vi "Check_Test_Voltage_and_Adjust.vi"(8 "error in":errorcluster, 11 "Voltage Desired":dbl format="%.6g") -> (0 "error out":errorcluster, 2 "Adjusted Voltage":dbl format="%.6g", 5 "Voltage Adjusted":bool)   [LabVIEW 2020]
uses:
  <vilib>/express/express arith-compare/Formula/XNode/ExpressFormulaBlockNode.xnode
panel:
  out "Outer While":i32
  out "Inner While":i32
  in  "Sample 1":dbl format="%.6g"
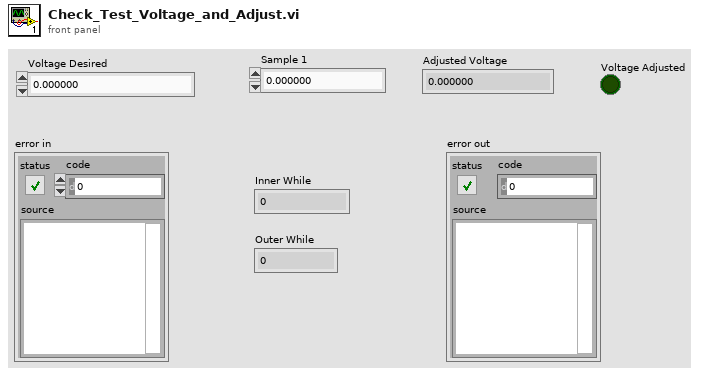
[diagram p1: front panel]
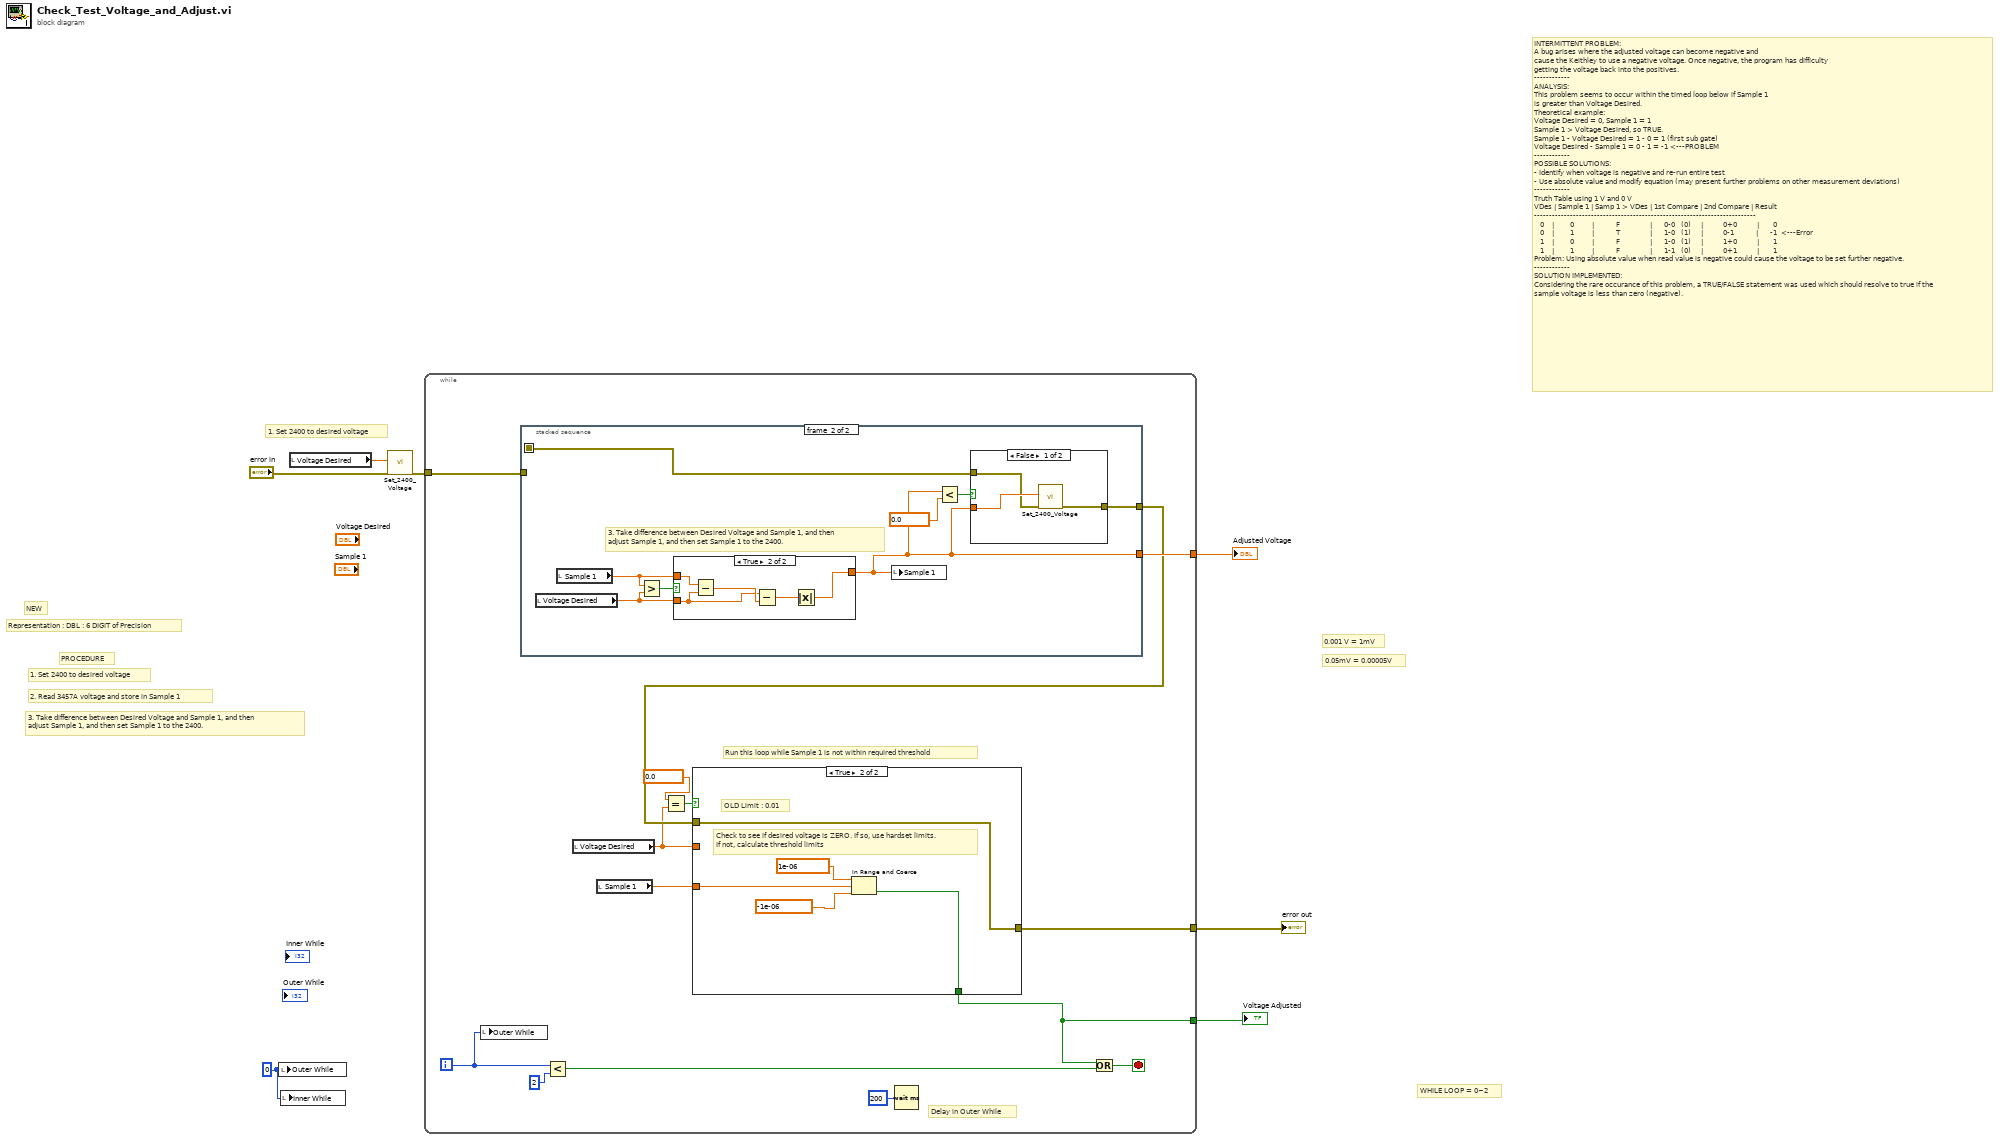
[diagram p0: block diagram]
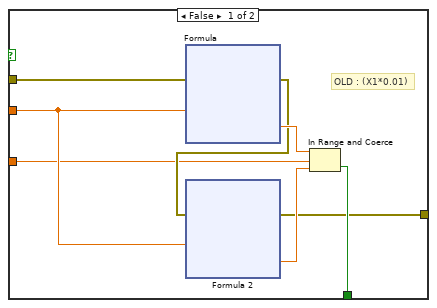
[diagram p2: hidden frame]
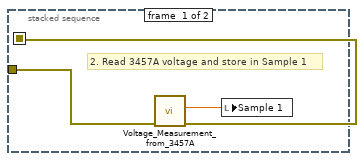
[diagram p3: hidden frame]
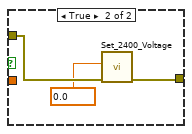
[diagram p4: hidden frame]
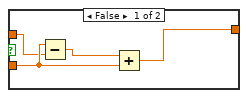
[diagram p5: hidden frame]
diagram:
  w1 = 0 ("Outer While")
  # "WHILE LOOP = 0~2"
  # "3. Take difference between Desired Voltage and Sample 1, and then\nadjust Sample 1, and then set Sample 1 to the 2400."
  # "NEW"
  # "2. Read 3457A voltage and store in Sample 1"
  # "Representation : DBL : 6 DIGIT of Precision"
  # "PROCEDURE"
  # "1. Set 2400 to desired voltage"
  # "0.05mV = 0.00005V"
  # "0.001 V = 1mV"
  # "INTERMITTENT PROBLEM:\nA bug arises where the adjusted voltage can become negative and\ncause the Keithley to use a negative voltage. Once negative, the program has difficulty \ngetting the voltage back into the positives.\n------------\nANALYSIS:\nThis problem seems to occur within the timed loop below if Sample 1\nis greater than Voltage Desired.\nTheoretical example:\nVoltage Desired = 0, Sample 1 = 1\nSample 1 > Voltage Desired, so TRUE.\nSample 1 - Voltage Desired = 1 - 0 = 1 (first sub gate)\nVoltage Desired - Sample 1 = 0 - 1 = -1 <---PROBLEM\n------------\nPOSSIBLE SOLUTIONS:\n- Identify when voltage is negative and re-run entire test\n- Use absolute value and modify equation (may present further problems on other measurement deviations)\n------------\nTruth Table using 1 V and 0 V\nVDes | Sample 1 | Samp 1 > VDes | 1st Compare | 2nd Compare | Result\n--------------------------------------------------------------------------\n   0    |        0         |           F               |      0-0   (0)     |          0+0          |       0\n   0    |        1         |           T               |      1-0   (1)     |          0-1           |      -1  <---Error\n   1    |        0         |           F               |      1-0   (1)     |          1+0          |       1\n   1    |        1         |           F               |      1-1   (0)     |          0+1          |       1\nProblem: Using absolute value when read value is negative could cause the voltage to be set further negative.\n------------\nSOLUTION IMPLEMENTED:\nConsidering the rare occurance of this problem, a TRUE/FALSE statement was used which should resolve to true if the sample voltage is less than zero (negative)."
  # "1. Set 2400 to desired voltage"
  n1 = local write "Outer While"(w1) -> ()
  n2 = local write "Inner While"(w1) -> ()
  n3 = local read "Voltage Desired"() -> (w2:dbl)
  n4 = call "Set_2400_Voltage.vi"("error in"="error in", "Voltage"=w2) -> ("error out"=w3:errorcluster)  [unwired: 8 in]
  n5 = while {
    tunnel: w3 -> [w16]
    tunnel: [w21] -> w7
    tunnel: [w9] -> w6
    tunnel: [w17] -> w5
    i -> [w8]
    stop <- w19 stop-if-true
    # "Delay in Outer While"
    # "Run this loop while Sample 1 is not within required threshold"
    n6 = local write "Outer While"(w8) -> ()
    n7 = stacked-sequence {
      seq-local: [w51 _] -> [_ w54]
      tunnel: [_ w56] -> w17
      tunnel: w16 -> [w52 _]
      tunnel: [_ w55] -> w15
      frame #0 {
        # "2. Read 3457A voltage and store in Sample 1"
        n8 = call "Voltage_Measurement_from_3457A.vi"("error in"=w52) -> ("error out"=w51:errorcluster, "mean"=w53:dbl)  [unwired: 9 in]
        n9 = local write "Sample 1"(w53) -> ()
      }
      frame #1 {
        # "3. Take difference between Desired Voltage and Sample 1, and then\nadjust Sample 1, and then set Sample 1 to the 2400."
        n10 = local read "Voltage Desired"() -> (w59:dbl)
        n11 = local read "Sample 1"() -> (w60:dbl)
        n12 = Greater?(x=w60, y=w59) -> (0:w61:bool)
        n13 = case shown="True" w61 {
          tunnel: w60 -> [w70 w75]
          tunnel: w59 -> [w71 w74]
          tunnel: [w68 w72] -> w56
          frame False {
            n14 = Subtract(x=w71, y=w70) -> (x-y=w69:dbl)
            n15 = Add(x=w69, y=w71) -> (x+y=w68:dbl)
          }
          frame True {
            n16 = Subtract(x=w75, y=w74) -> (x-y=w76:dbl)
            n17 = Subtract(x=w74, y=w76) -> (x-y=w73:dbl)
            n18 = Absolute Value(x=w73) -> (abs(x)=w72:dbl)
          }
        }
        n19 = local write "Sample 1"(w56) -> ()
        n20 = Less?(x=w56, y=0.0) -> (x < y?=w57:bool)
        n21 = case shown="False" w57 {
          tunnel: w56 -> [w64 _]
          tunnel: w54 -> [w63 w67]
          tunnel: [w62 w66] -> w55
          frame False {
            n22 = call "Set_2400_Voltage.vi"("error in"=w63, "Voltage"=w64) -> ("error out"=w62:errorcluster)  [unwired: 8 in]
          }
          frame True {
            n23 = call "Set_2400_Voltage.vi"("error in"=w67, "Voltage"=0.0 ("y")) -> ("error out"=w66:errorcluster)  [unwired: 8 in]
          }
        }
      }
    }
    n24 = Less?(x=w8, y=2) -> (x < y?=w18:bool)
    n25 = local read "Voltage Desired"() -> (w12:dbl)
    n26 = local read "Sample 1"() -> (w11:dbl)
    n27 = Equal?(x=0.0 ("y"), y=w12) -> (x = y?=w13:bool)
    n28 = case shown="True" w13 {
      tunnel: [w26 w49] -> w9
      tunnel: w12 -> [w25 _]
      tunnel: w11 -> [w24 w50]
      tunnel: w15 -> [w23 w48]
      tunnel: [w22 w48] -> w21
      frame False {
        # "OLD : (X1*0.01)"
        n29 = xnode ("Formula")("X1"=w25, "error in (no error)"=w23) -> ("Result"=w29:dbl, "error out"=w27:errorcluster)
        n30 = xnode ("Formula 2")("X1"=w25, "error in (no error)"=w27) -> ("Result"=w28:dbl, "error out"=w22:errorcluster)
        n31 = In Range and Coerce(upper limit=w29, x=w24, lower limit=w28) -> (In Range?=w26:bool)  [unwired: 1 out]
      }
      frame True {
        # "OLD Limit : 0.01"
        # "Check to see if desired voltage is ZERO. If so, use hardset limits.\nIf not, calculate threshold limits"
        n32 = In Range and Coerce(upper limit=1e-06 ("y"), x=w50, lower limit=-1e-06 ("y")) -> (In Range?=w49:bool)  [unwired: 1 out]
      }
    }
    n33 = Wait (ms)(milliseconds to wait=u32 200) -> ()  [unwired: 1 out]
    n34 = Or(x=w9, y=w18) -> (x .or. y?=w19:bool)
  }
  "error out" <- w7
  "Voltage Adjusted" <- w6
  "Adjusted Voltage" <- w5
